vi "Delacor_lib_QMH_Set Error Debug.vi"(8 "error in":errorcluster, 10 "Error Debug":string, 11 "Message Queue in":refnum<class "Delacor_lib_QMH_Message Queue.lvclass">) -> (0 "error out":errorcluster, 3 "Message Queue out":refnum<class "Delacor_lib_QMH_Message Queue.lvclass">)   [LabVIEW 2024, in "Delacor_lib_QMH_Message Queue.lvclass"]
doc: "____\nDQMH Framework: Palette 7.1.0.1503\nCopyright (c) 2025, DQMH Consortium"
uses:
  Delacor_lib_QMH_Message Queue.lvclass
  Delacor_lib_QMH_Message Queue.lvclass/Delacor_lib_QMH_Message Queue.ctl
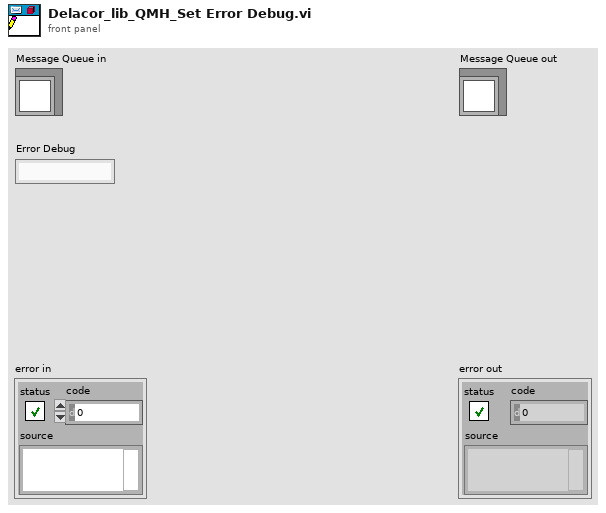
[diagram p1: front panel]
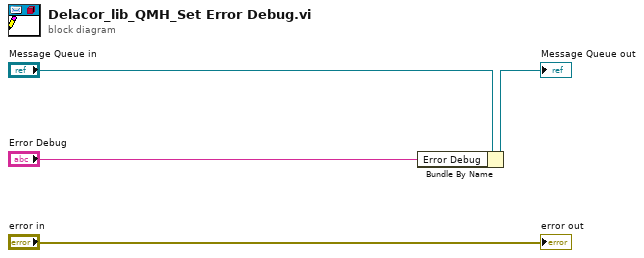
[diagram p0: block diagram]
diagram:
  n1 = Bundle By Name(cluster="Message Queue in", "Error Debug"="Error Debug") -> (→"Message Queue out":refnum<class "Delacor_lib_QMH_Message Queue.lvclass">)
  "error out" <- "error in"
